vi "20170509-lecture4-1 runtime menu.vi"() -> ()   [LabVIEW 2014]
panel:
  in  "stop":bool
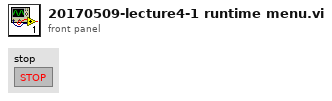
[diagram p1: front panel]
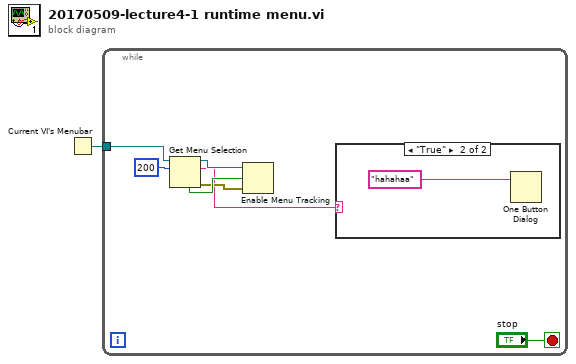
[diagram p0: block diagram]
diagram:
  n1 = Current VI's Menubar() -> (w1:refnum<k9>)
  n2 = while {
    tunnel: w1 -> [w5]
    stop <- "stop" stop-if-true
    n3 = Get Menu Selection(0:w5, 1:200 ("ms timeout (200)")) -> (4:w8:bool, 5:w7:refnum<k9>, 6:w3:string, 8:w6:errorcluster)  [unwired: 2 in, 1 out]
    n4 = Enable Menu Tracking(2:w6, 3:w8, 4:w7) -> ()  [unwired: 2 out]
    n5 = case shown="\"True\"" w3 {
      frame "False", Default {
      }
      frame "True" {
        n6 = One Button Dialog(message="hahahaa") -> ()  [unwired: 1 in, 1 out]
      }
    }
  }
